vi "MTU Chip Corner Get Corner.vi"(9 "Param":T3={"Select Mode \n0: Dark\n1: light"=1.0, "Threshold Value"=200.0, "Chip Long Side Size"=25.0, "Chip Long Side Min Tolerance"=0.8, "Chip Long Side Max Tolerance"=1.5, "Chip Short Side Size"=15.0, "Chip Short Side Min Tolerance"=0.8, "Chip Short Side Max Tolerance"=1.5, "Chip Pitch X"=70.0, "Chip Pitch Y"=70.0, "Edge Exclusion Distance"=200.0, "Reserve[11]"=0.0, "Reserve[12]"=0.0, "Parameters[13]"=0.0, "Parameters[14]"=0.0, "Parameters[15]"=0.0, "Parameters[16]"=0.0, "Parameters[17]"=0.0, "Parameters[18]"=0.0, "Parameters[19]"=0.0}) -> (1 "fPosX":sgl[](array[numeric]), 2 "boolResult":sgl[](array[numeric]), 4 "fAngle":sgl[](array[numeric]), 5 "fPosY":sgl[](array[numeric]))   [LabVIEW 2017, in "AOILib_MTUchipcorner_V1.lvlib"]
doc: "__declspec(dllexport) void MTUChipCorner_GetCorner(unsigned int* imageIN, ImgP imageParm, paramChipCorner Param,\n unsigned int* imageOUT, float boolResult[], float fPosX[], float fPosY[], float fAngle[]);"
uses:
  <userlib>/AOILib_MTUchipcorner_V1/AOILib_MTUchipcorner_V1.lvlib
  <vilib>/vision/NI_Vision_Development_Module.lvlib
panel:
  out "image out":T1(plugin-control)
  in  "File Path_IMGin":path=path "C:/Users/MyUser/Desktop/Harvie Test/CornerChip/ChipCornerTest.bmp"
  out "image":T1(plugin-control)
  out "X Resolution":i32
  out "Y Resolution":i32
  in  "imageParm 2":T2={"PICmode"=0, "Outputmode"=0, "cols"=2448, "rows"=2048, "correctTheta"=0.0}
  out "error out":errorcluster
  # "boolResult[0] 列表\n\n0:中間過渡 (理論上不應該出現 出現 0 代表有BUG)\n1:無法找到足夠數量的Chip識別Corner Chip,請確認是否有拍到Chip\n或者影像亮暗需要調整\n2:目前拍照位置 Chip分布 無法被判斷成角點 Corner Chip\n9:正常檢出角點並取得角度"
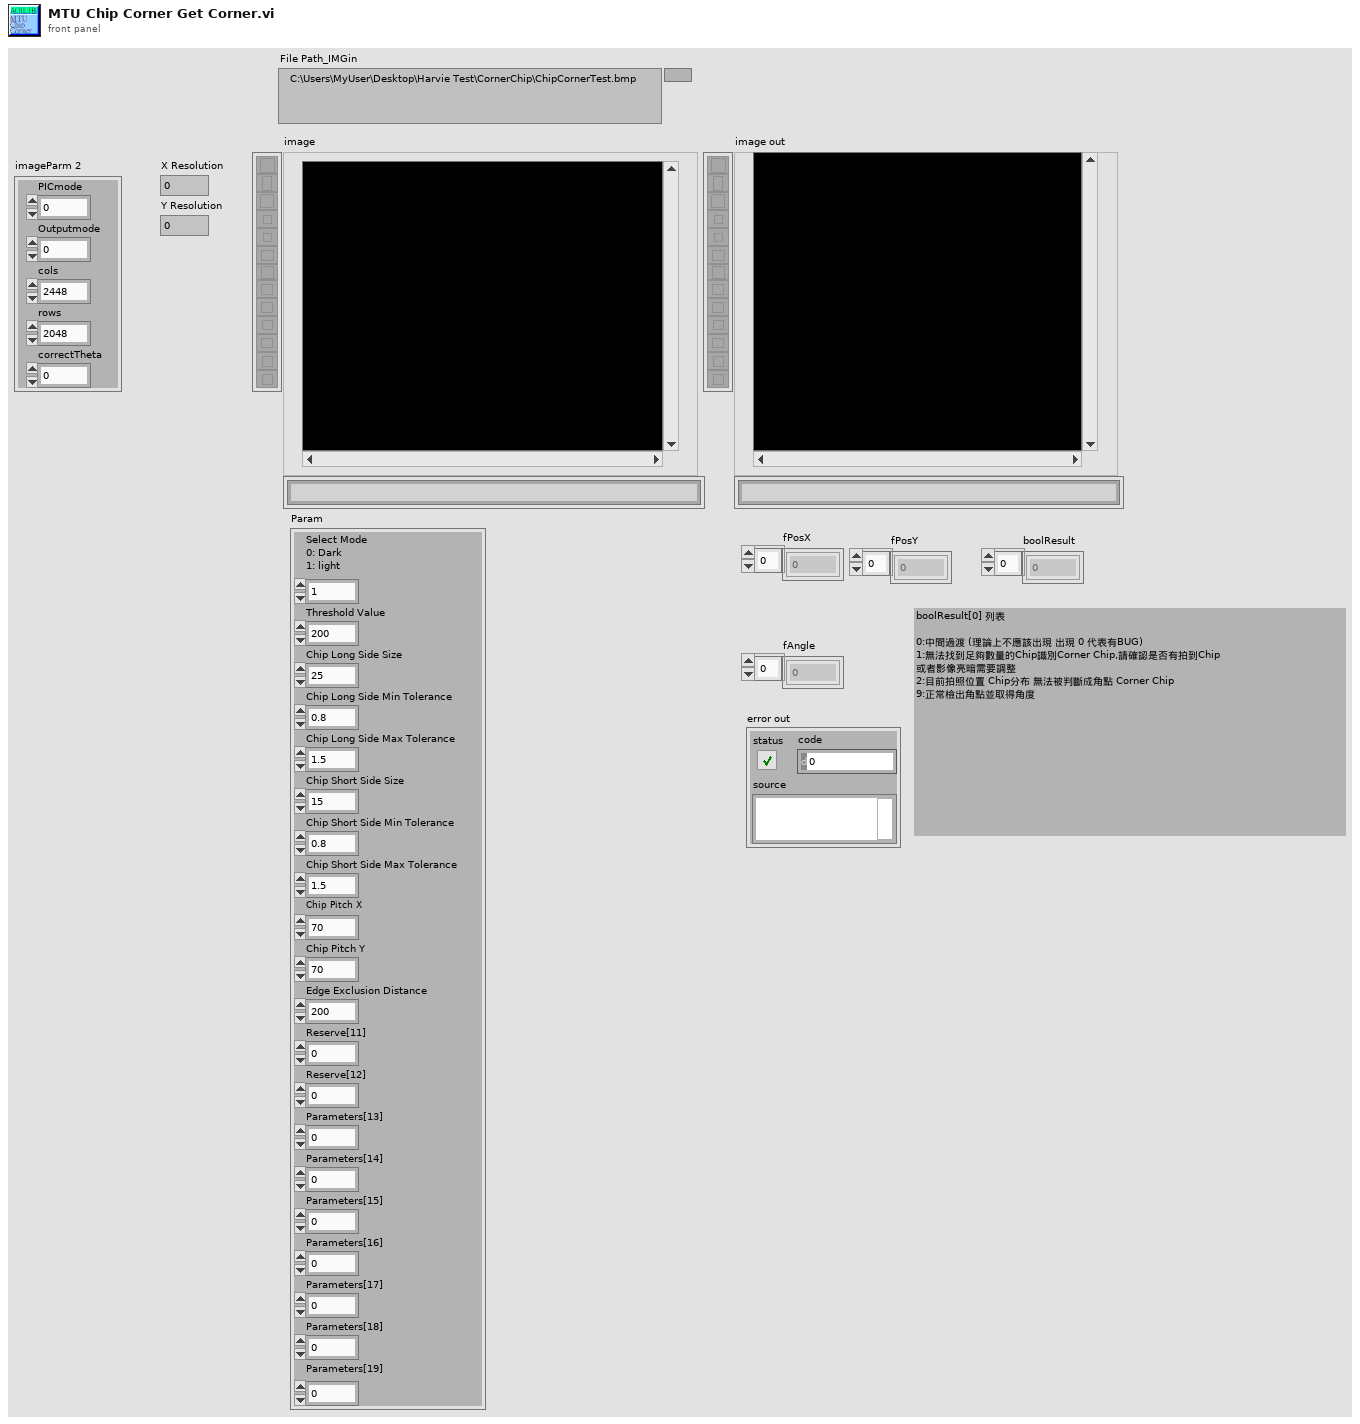
[diagram p1: front panel]
types:
  T1 = typedef "IMAQ Image.ctl" = refnum<image>
  T2 = cluster{"PICmode":i32, "Outputmode":i32, "cols":i32, "rows":i32, "correctTheta":dbl}
  T3 = cluster{"Select Mode \n0: Dark\n1: light":sgl, "Threshold Value":sgl, "Chip Long Side Size":sgl, "Chip Long Side Min Tolerance":sgl, "Chip Long Side Max Tolerance":sgl, "Chip Short Side Size":sgl, "Chip Short Side Min Tolerance":sgl, "Chip Short Side Max Tolerance":sgl, "Chip Pitch X":sgl, "Chip Pitch Y":sgl, "Edge Exclusion Distance":sgl, "Reserve[11]":sgl, "Reserve[12]":sgl, "Parameters[13]":sgl, "Parameters[14]":sgl, "Parameters[15]":sgl, "Parameters[16]":sgl, "Parameters[17]":sgl, "Parameters[18]":sgl, "Parameters[19]":sgl}
  T4 = typedef "Image Type" = u32
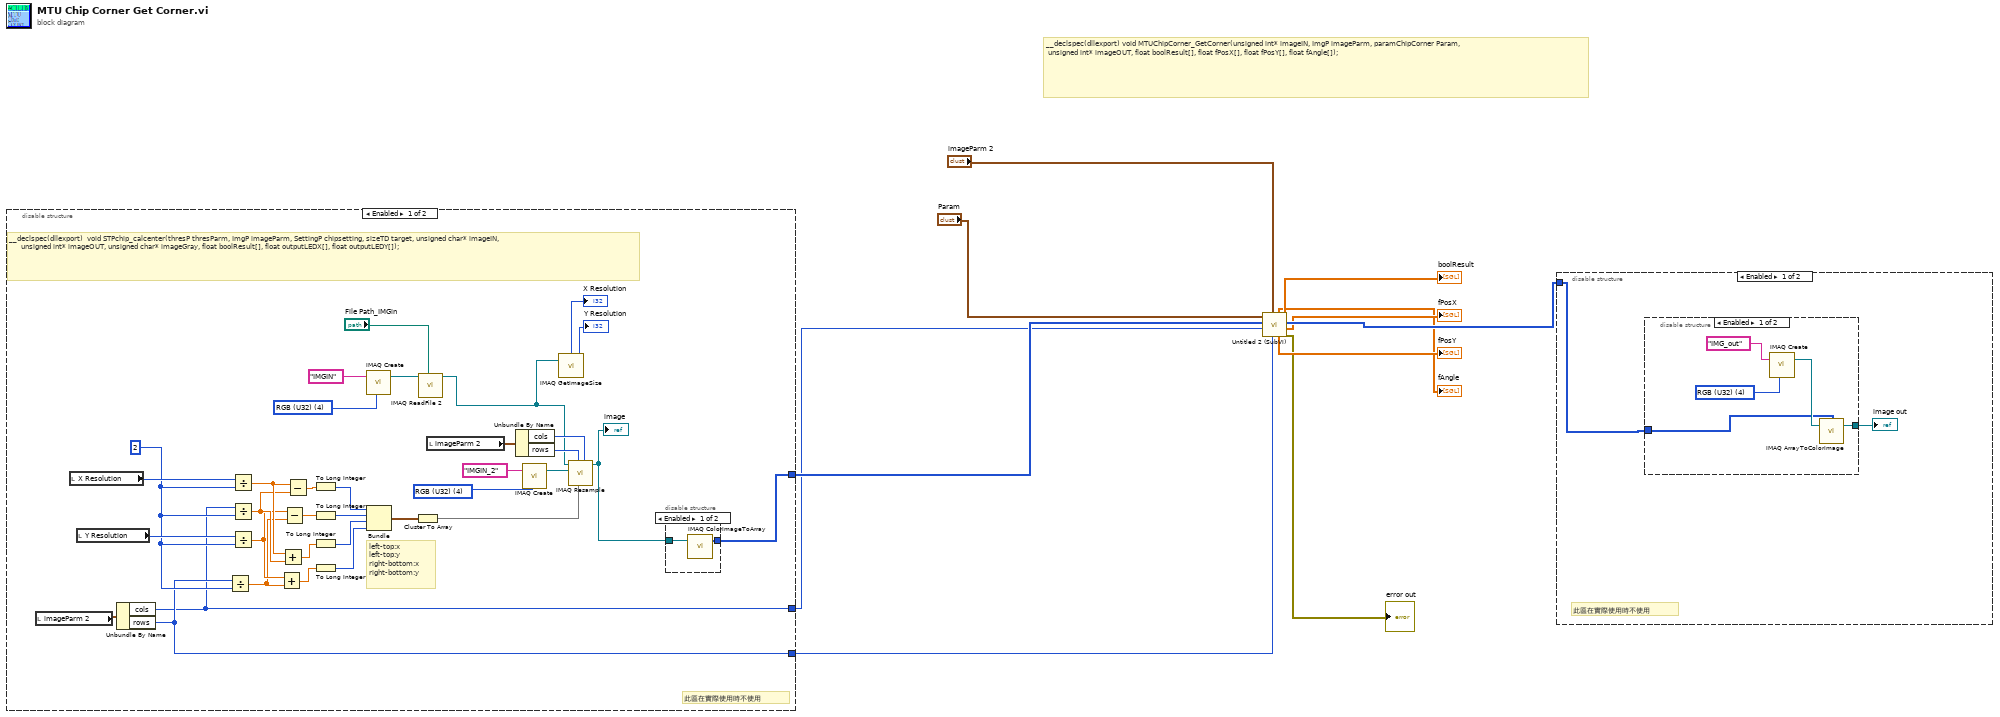
[diagram p0: block diagram]
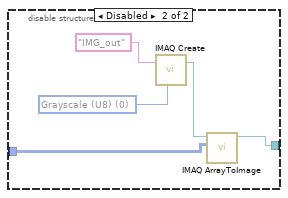
[diagram p2: hidden frame]
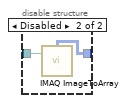
[diagram p4: hidden frame]
diagram:
  # "__declspec(dllexport) void MTUChipCorner_GetCorner(unsigned int* imageIN, ImgP imageParm, paramChipCorner Param,\n\tunsigned int* imageOUT, float boolResult[], float fPosX[], float fPosY[], float fAngle[]);"
  n1 = disable-structure shown="Enabled" {
    disable-tunnel: [w15 _] -> w10
    disable-tunnel: [w14 _] -> w7
    disable-tunnel: [w13 _] -> w6
    frame Enabled {
      w17 = T4 4 items=["Grayscale (U8)", "Grayscale (I16)", "Grayscale (SGL)", "Complex (CSG)", "RGB (U32)", "HSL (U32)", "RGB (U64)", "Grayscale (U16)"] ("Image Type")
      w18 = T4 4 items=["Grayscale (U8)", "Grayscale (I16)", "Grayscale (SGL)", "Complex (CSG)", "RGB (U32)", "HSL (U32)", "RGB (U64)", "Grayscale (U16)"] ("Image Type")
      w33 = 2 ("y")
      # "__declspec(dllexport)  void STPchip_calcenter(thresP thresParm, ImgP imageParm, SettingP chipsetting, sizeTD target, unsigned char* imageIN,\n\t\t\t\t\t\tunsigned int* imageOUT, unsigned char* imageGray, float boolResult[], float outputLEDX[], float outputLEDY[]);"
      # "此區在實際使用時不使用"
      # "left-top:x\nleft-top:y\nright-bottom:x\nright-bottom:y"
      n2 = local read "imageParm 2"() -> (w39:T2)
      n3 = local read "X Resolution"() -> (w35:i32)
      n4 = local read "Y Resolution"() -> (w34:i32)
      n5 = Unbundle By Name(w39) -> ("cols"=w13:i32, "rows"=w14:i32)
      n6 = Divide(x=w14, y=w33) -> (x/y=w26:dbl)
      n7 = Divide(x=w35, y=w33) -> (x/y=w30:dbl)
      n8 = Divide(x=w13, y=w33) -> (x/y=w29:dbl)
      n9 = Divide(x=w34, y=w33) -> (x/y=w27:dbl)
      n10 = Add(x=w27, y=w26) -> (x+y=w25:dbl)
      n11 = Add(x=w30, y=w29) -> (x+y=w28:dbl)
      n12 = Subtract(x=w27, y=w26) -> (x-y=w31:dbl)
      n13 = Subtract(x=w30, y=w29) -> (x-y=w32:dbl)
      n14 = To Long Integer(number=w32) -> (32bit integer=w24:i32)
      n15 = To Long Integer(number=w31) -> (32bit integer=w23:i32)
      n16 = To Long Integer(number=w28) -> (32bit integer=w22:i32)
      n17 = To Long Integer(number=w25) -> (32bit integer=w21:i32)
      n18 = call "IMAQ Create"("Image Name"="IMGIN", "Image Type"=w18) -> ("New Image"=w45:T1)  [unwired: 3 in, 1 out]
      n19 = Bundle(w24, w23, w22, w21) -> (w20:cluster{i32, i32, i32, i32})  [unwired: 1 in]
      n20 = Cluster To Array(cluster=w20) -> (array=w19:i32[])
      n21 = call "IMAQ ReadFile 2"("File Path"="File Path_IMGin", "Image"=w45) -> ("Image Out"=w16:T1)  [unwired: 5 in, 4 out]
      n22 = local read "imageParm 2"() -> (w42:T2)
      n23 = Unbundle By Name(w42) -> ("cols"=w41:i32, "rows"=w40:i32)
      n24 = call "IMAQ Create"("Image Name"="IMGIN_2", "Image Type"=w17) -> ("New Image"=w38:T1)  [unwired: 3 in, 1 out]
      n25 = call "IMAQ GetImageSize"("Image"=w16) -> ("Y Resolution"=→"Y Resolution":i32, "X Resolution"=→"X Resolution":i32)  [unwired: 3 in, 1 out]
      n26 = call "IMAQ Resample"("X Resolution"=w41, "Optional Rectangle"=w19, "Y Resolution"=w40, "Image Dst"=w38, "Image Src"=w16) -> ("Image Dst Out"=w12:T1)  [unwired: 5 in, 1 out]
      "image" <- w12
      n27 = disable-structure shown="Enabled" {
        disable-tunnel: w12 -> [w48 w50]
        disable-tunnel: [w47 w49] -> w15
        frame Enabled {
          n28 = call "IMAQ ColorImageToArray"("Image"=w48) -> ("Image Pixels (U32)"=w47:u32[][])  [unwired: 3 in, 2 out]
        }
        frame Disabled {
          n29 = call "IMAQ ImageToArray"("Image"=w50) -> ("Image Pixels (U8)"=w49:u8[][])  [unwired: 3 in, 4 out]
        }
      }
    }
    frame Disabled {
    }
  }
  n30 = call <userlib>:"Untitled 2 (SubVI).vi"("rows"=w7, "imageParm in"="imageParm 2", "cols"=w6, "Image Pixels (U32)"=w10, "Param"="Param") -> ("error out"=→"error out":errorcluster, "fPosX"=→"fPosX":sgl[], "imageOUT"=w8:u32[][], "boolResult"=→"boolResult":sgl[], "fPosY"=→"fPosY":sgl[], "fAngle"=→"fAngle":sgl[])  [unwired: 1 in]
  n31 = disable-structure shown="Enabled" {
    disable-tunnel: w8 -> [w51 _]
    frame Enabled {
      # "此區在實際使用時不使用"
      n32 = disable-structure shown="Enabled" {
        disable-tunnel: [w56 w61] -> w52
        disable-tunnel: w51 -> [w53 w60]
        frame Enabled {
          w54 = T4 4 items=["Grayscale (U8)", "Grayscale (I16)", "Grayscale (SGL)", "Complex (CSG)", "RGB (U32)", "HSL (U32)", "RGB (U64)", "Grayscale (U16)"] ("Image Type")
          n33 = call "IMAQ Create"("Image Name"="IMG_out", "Image Type"=w54) -> ("New Image"=w57:T1)  [unwired: 3 in, 1 out]
          n34 = call "IMAQ ArrayToColorImage"("Image Pixels (U32)"=w53, "Image"=w57) -> ("Image Out"=w56:T1)  [unwired: 3 in, 1 out]
        }
        frame Disabled {
          w62 = T4 0 items=["Grayscale (U8)", "Grayscale (I16)", "Grayscale (SGL)", "Complex (CSG)", "RGB (U32)", "HSL (U32)", "RGB (U64)", "Grayscale (U16)"] ("Image Type")
          n35 = call "IMAQ Create"("Image Name"="IMG_out", "Image Type"=w62) -> ("New Image"=w58:T1)  [unwired: 3 in, 1 out]
          n36 = call "IMAQ ArrayToImage"("Image Pixels (U8)"=w60, "Image"=w58) -> ("Image Out"=w61:T1)  [unwired: 8 in, 1 out]
        }
      }
      "image out" <- w52
    }
    frame Disabled {
    }
  }
